vi "Create Arbitrary Waveform_Corr1.vi"(6 "Arbitrary Numeric Waveform Data":dbl[](array[numeric])=[1000.0, 2000.0, 3000.0, 4000.0, 5000.0, 6000.0, 7000.0, 8000.0], 7 "Waveform Parameters":T1={"Frequency (1000 Hz)"=1000.0, "Amplitude (2.0 Vpp)"=2.0, "DC Offset (0.00 V)"=0.0, "Phase (0.0 degrees)"=0.002} {"Phase (0.0 degrees)" min=-360.0 max=360.0 format="%#.1g"; "DC Offset (0.00 V)" min=-10.0 max=10.0; "Amplitude (2.0 Vpp)" min=0.001 max=20.0 step=1.0 format="%#.3f"; "Frequency (1000 Hz)" min=1e-06 max=160000000.0 step=1.0 format="%#.6g"}, 8 "error in (no error)":errorcluster, 9 "Select Channel (1:Channel 1)":i32(ring)=1 items=["Channel 1"=1, "Channel 2"=2], 10 "Waveform Name (\"wave1\")":string="wave1", 11 "VISA resource name":refnum<visa-resource-name>="USB0::0xF4EC::0x1101::SDG6XEBC5R0119::INSTR") -> (0 "error out":errorcluster, 3 "VISA resource name out":refnum<visa-resource-name>)   [LabVIEW 2018]
doc: "Creates and saves an arbitrary (user-defined) waveform in non-volatile memory, then selects it for output."
panel:
  # "Same vi as with suppliers example,\nbut incorrect negativ case removed.\nInstead calculating twos complement\nexplicitly for negative values.\nThe input range for ARB data is\n-32768..+32767"
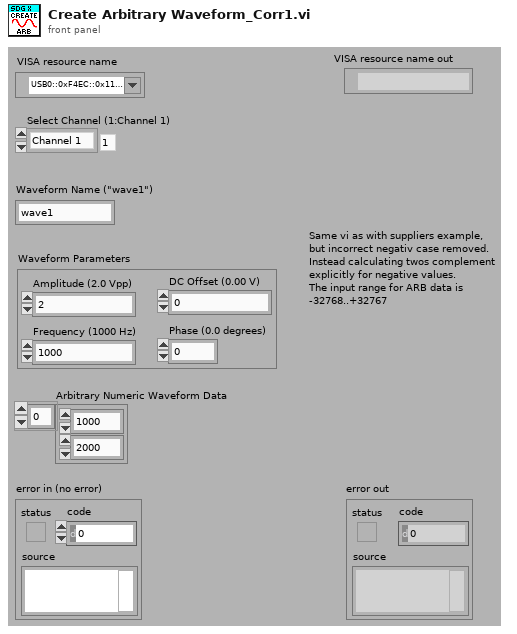
[diagram p1: front panel]
types:
  T1 = cluster{"Frequency (1000 Hz)":dbl, "Amplitude (2.0 Vpp)":dbl, "DC Offset (0.00 V)":dbl, "Phase (0.0 degrees)":dbl}
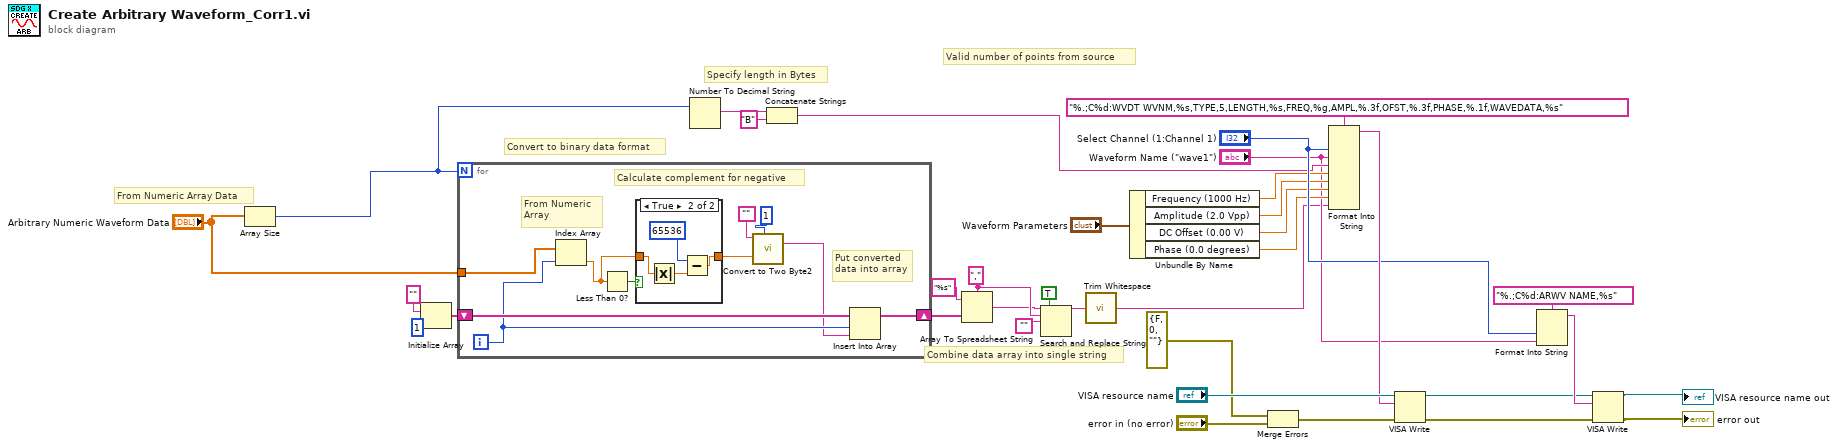
[diagram p0: block diagram]
diagram:
  w20 = ","
  # "From Numeric Array Data"
  # "Specify length in Bytes"
  # "Combine data array into single string"
  # "Valid number of points from source"
  # "Convert to binary data format"
  n1 = Array Size(array="Arbitrary Numeric Waveform Data") -> (size(s)=w28:i32)
  n2 = Initialize Array("", 1) -> (w24:string[])
  n3 = for {
    N: w28 -> [_]
    tunnel: "Arbitrary Numeric Waveform Data" -> [w43]
    shift-right: [w39] -> w5
    shift-left: w24 -> [w42]
    i -> [w41]
    # "Calculate complement for negative"
    # "From Numeric\nArray"
    # "Put converted\ndata into array"
    n4 = Index Array(array=w43, index=w41) -> (element=w37:dbl)
    n5 = Less Than 0?(x=w37) -> (x < 0?=w38:bool)
    n6 = case shown="True" w38 {
      tunnel: w37 -> [w46 w47]
      tunnel: [w46 w50] -> w36
      frame False {
      }
      frame True {
        n7 = Absolute Value(x=w47) -> (abs(x)=w48:dbl)
        n8 = Subtract(x=65536, y=w48) -> (x-y=w50:dbl)
      }
    }
    n9 = call "Convert to Two Byte2.vi"("Input Method (0:String)"=u16 1, "Input Number"=w36, "Numeric String"="") -> ("Output String"=w40:string)  [unwired: 8 in]
    n10 = Insert Into Array(array=w42, index=w41, new element=w40) -> (w39:string[])
  }
  n11 = Number To Decimal String(number=w28) -> (decimal integer string=w14:string)  [unwired: 1 in]
  n12 = Concatenate Strings(w14, "B" ("string")) -> (w12:string)
  n13 = Array To Spreadsheet String(delimiter (Tab)=w20, array=w5, 3:"%s") -> (spreadsheet string=w17:string)
  n14 = Search and Replace String(replace all?=TRUE, input string=w17, search string=w20, replace string="") -> (result string=w18:string)  [unwired: 4 in, 3 out]
  n15 = call <vilib>:"Trim Whitespace.vi"("string"=w18) -> ("trimmed string"=w6:string)  [unwired: 1 in]
  n16 = Unbundle By Name("Waveform Parameters") -> ("Frequency (1000 Hz)"=w11:dbl, "Amplitude (2.0 Vpp)"=w10:dbl, "DC Offset (0.00 V)"=w9:dbl, "Phase (0.0 degrees)"=w8:dbl)
  n17 = Merge Errors(errorcluster {"status"=FALSE, "code"=0, "source"=""} ("error constant"), "error in (no error)") -> (w30:errorcluster)
  n18 = Format Into String(format string="%.;C%d:WVDT WVNM,%s,TYPE,5,LENGTH,%s,FREQ,%g,AMPL,%.3f,OFST,%.3f,PHASE,%.1f,WAVEDATA,%s", "Select Channel (1:Channel 1)", "Waveform Name (\"wave1\")", w12, w11, w10, w9, w8, w6) -> (resulting string=w33:string)  [unwired: 2 in, 1 out]
  n19 = VISA Write(VISA resource name="VISA resource name", write buffer=w33, error in (no error)=w30) -> (VISA resource name out=w4:refnum<visa-resource-name>, error out=w3:errorcluster)  [unwired: 1 out]
  n20 = Format Into String(format string="%.;C%d:ARWV NAME,%s", "Select Channel (1:Channel 1)", "Waveform Name (\"wave1\")") -> (resulting string=w29:string)  [unwired: 2 in, 1 out]
  n21 = VISA Write(VISA resource name=w4, write buffer=w29, error in (no error)=w3) -> (VISA resource name out=→"VISA resource name out":refnum<visa-resource-name>, error out=→"error out":errorcluster)  [unwired: 1 out]
